vi "conditional_off.vi"(4 "switch off?":bool, 5 "boolean in":bool) -> (1 "boolean out":bool)   [LabVIEW 2010]
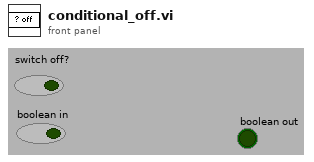
[diagram p1: front panel]
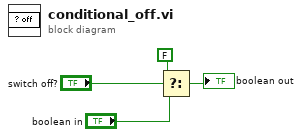
[diagram p0: block diagram]
diagram:
  n1 = Select(t=FALSE, s="switch off?", f="boolean in") -> (s? t:f=→"boolean out":bool)
